vi "NXT_MIDBRAIN Get Max Index.vi"(1 "Array":i8[](array[numeric]), 2 "_motorCommands":T1={"_rudderCommand"=7, "_propCommand"=7, "_irServoCommand"=7}) -> (0 "Max Index":i8)   [LabVIEW 2012, in "Tugboat.lvrbt"]
uses:
  Tugboat.lvrbt
  motorCommands_t.ctl
panel:
  out "element":i8
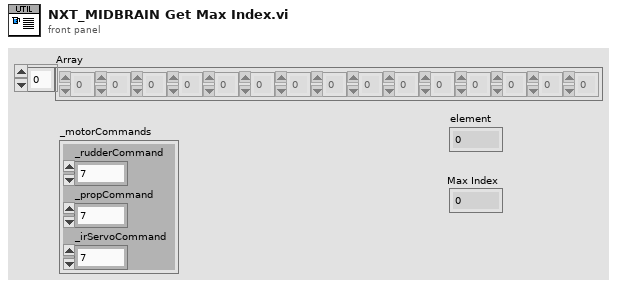
[diagram p1: front panel]
types:
  T1 = typedef "motorCommands_t.ctl" = cluster{"_rudderCommand":i8, "_propCommand":i8, "_irServoCommand":i8}
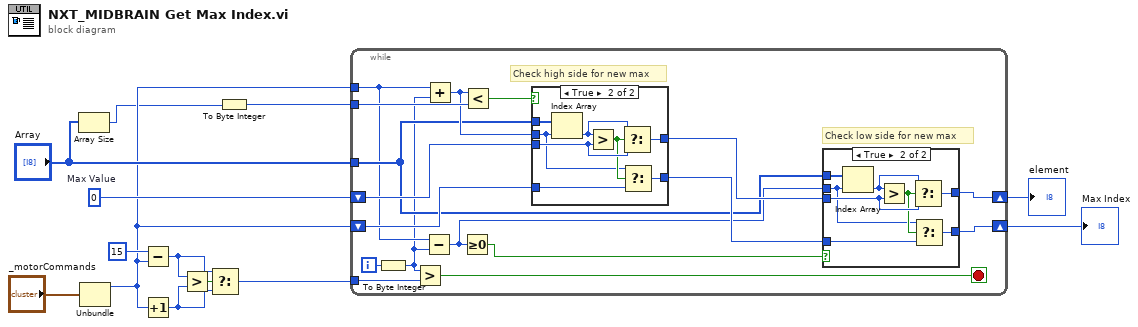
[diagram p0: block diagram]
diagram:
  w7 = i8 0  # Max Value
  n1 = Array Size(array="Array") -> (size(s)=w2:i32)
  n2 = Unbundle("_motorCommands") -> ("_rudderCommand"=w5:i8)  [unwired: 2 out]
  n3 = Subtract(x=i8 15, y=w5) -> (x-y=w10:i8)
  n4 = Increment(x=w5) -> (x+1=w9:i8)
  n5 = Greater?(x=w10, y=w9) -> (0:w11:bool)
  n6 = Select(t=w10, s=w11, f=w9) -> (s? t:f=w8:i8)
  n7 = To Byte Integer(number=w2) -> (8bit integer=w1:i8)
  n8 = while {
    tunnel: w8 -> [w30]
    tunnel: "Array" -> [w17]
    shift-right: [w21] -> w4
    shift-left: w7 -> [w25]
    shift-right: [w20] -> w3
    shift-left: w5 -> [w24]
    tunnel: w1 -> [w28]
    tunnel: w5 -> [w16]
    i -> [w15]
    stop <- w29 stop-if-true
    # "Check low side for new max"
    # "Check high side for new max"
    n9 = To Byte Integer(number=w15) -> (8bit integer=w14:i8)
    n10 = Greater?(x=w14, y=w30) -> (0:w29:bool)
    n11 = Subtract(x=w16, y=w14) -> (x-y=w18:i8)
    n12 = Add(x=w16, y=w14) -> (x+y=w26:i8)
    n13 = Greater Or Equal To 0?(x=w18) -> (x >= 0?=w19:bool)
    n14 = Less?(x=w26, y=w28) -> (x < y?=w27:bool)
    n15 = case shown="True" w27 {
      tunnel: w26 -> [_ w45]
      tunnel: w17 -> [_ w50]
      tunnel: w25 -> [w41 w48]
      tunnel: w24 -> [w42 w46]
      tunnel: [w41 w44] -> w22
      tunnel: [w42 w43] -> w23
      frame False {
      }
      frame True {
        n16 = Index Array(array=w50, index=w45) -> (element=w49:i8)
        n17 = Greater?(x=w49, y=w48) -> (0:w47:bool)
        n18 = Select(t=w49, s=w47, f=w48) -> (s? t:f=w44:i8)
        n19 = Select(t=w45, s=w47, f=w46) -> (s? t:f=w43:i8)
      }
    }
    n20 = case shown="True" w19 {
      tunnel: w18 -> [_ w35]
      tunnel: w17 -> [_ w40]
      tunnel: w22 -> [w31 w38]
      tunnel: w23 -> [w32 w36]
      tunnel: [w31 w34] -> w21
      tunnel: [w32 w33] -> w20
      frame False {
      }
      frame True {
        n21 = Index Array(array=w40, index=w35) -> (element=w39:i8)
        n22 = Greater?(x=w39, y=w38) -> (0:w37:bool)
        n23 = Select(t=w39, s=w37, f=w38) -> (s? t:f=w34:i8)
        n24 = Select(t=w35, s=w37, f=w36) -> (s? t:f=w33:i8)
      }
    }
  }
  "Max Index" <- w3
  "element" <- w4
